vi "Parse VTG Sentence.vi"(8 "error in (no error)":errorcluster, 11 "VTG sentence":string) -> (0 "error out":errorcluster, 3 "VTG  data":T1 {"type of fix"."mode" items=["Simulator", "Not Valid", "Estimated", "Differential", "Autonomous"]})   [LabVIEW 2017, in "NMEA API.lvlib"]
doc: "Returns data contained in a particular type of NMEA sentence. The input sentence you specify must include valid NMEA formatting and end with a carriage return and line feed, or \\r\\n. You must manually select the polymorphic instance to use."
uses:
  <vilib>/robotics/Protocols/NMEA/NMEA API.lvlib
  <vilib>/robotics/Protocols/NMEA/typedefs/VTG Data.ctl
  <vilib>/robotics/Utilities/NI_Robotics Utilities.lvlib
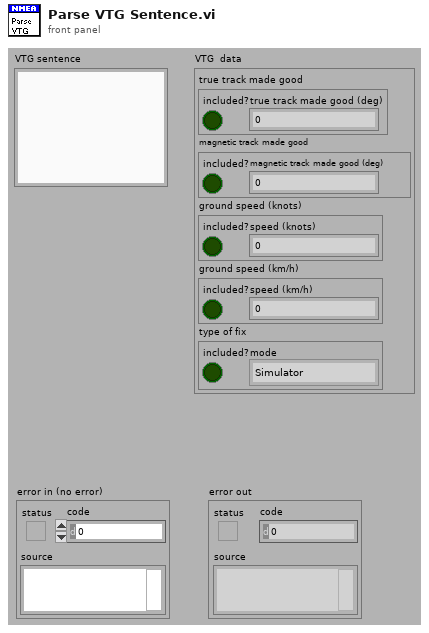
[diagram p1: front panel]
types:
  T1 = typedef "NMEA API.lvlib/VTG Data.ctl" = cluster{"true track made good":cluster{"included?":bool, "true track made good (deg)":dbl}, "magnetic track made good":cluster{"included?":bool, "magnetic track made good (deg)":dbl}, "ground speed (knots)":cluster{"included?":bool, "speed (knots)":dbl}, "ground speed (km/h)":cluster{"included?":bool, "speed (km/h)":dbl}, "type of fix":cluster{"included?":bool, "mode":u16}}
  T2 = cluster{"Boolean":bool, "True Track Made Good (Deg)":dbl}
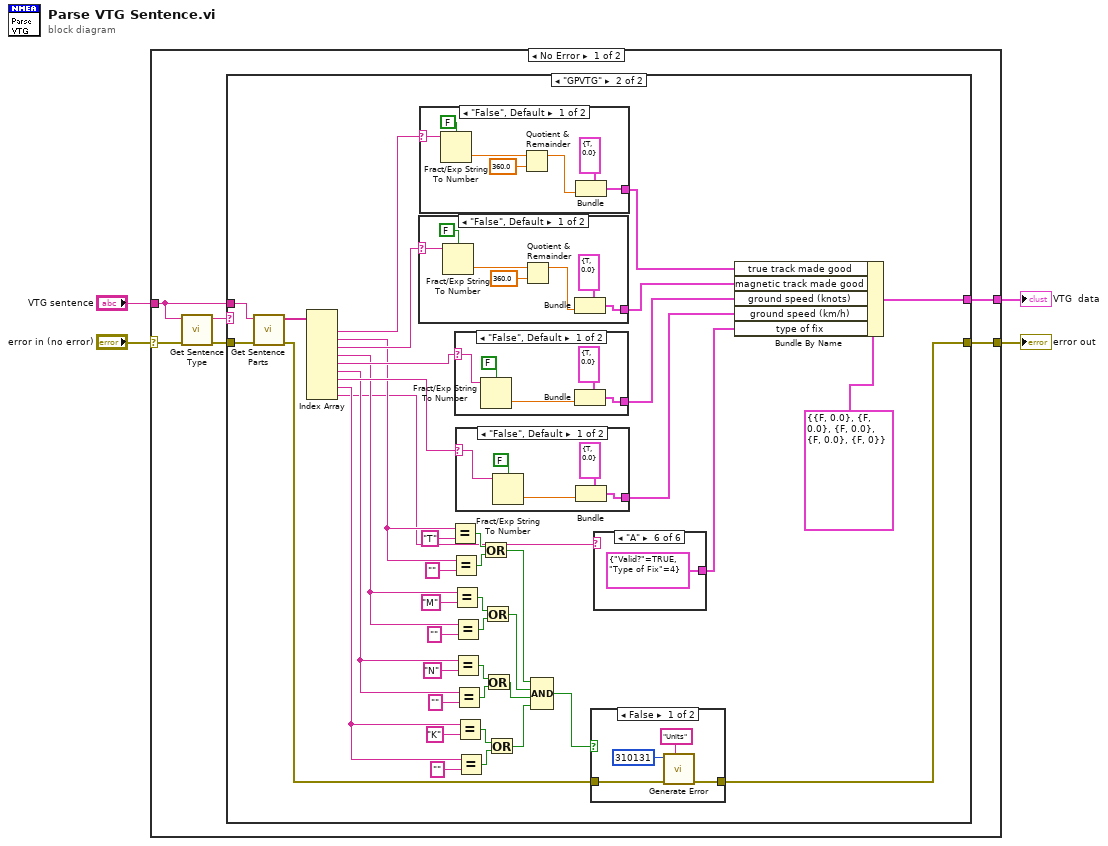
[diagram p0: block diagram]
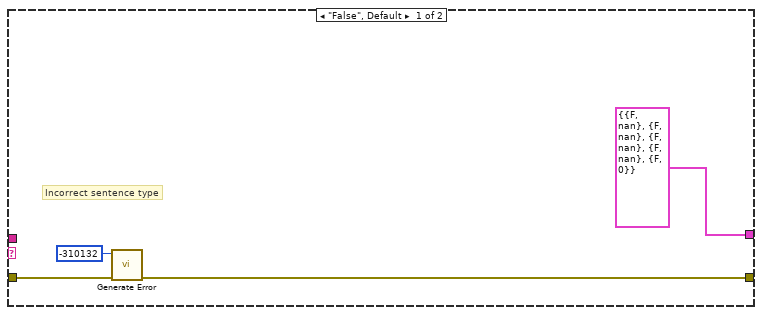
[diagram p2: hidden frame]
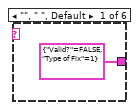
[diagram p3: hidden frame]
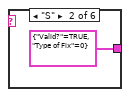
[diagram p4: hidden frame]
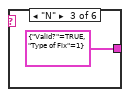
[diagram p5: hidden frame]
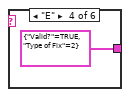
[diagram p6: hidden frame]
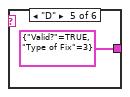
[diagram p7: hidden frame]
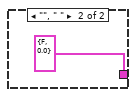
[diagram p9: hidden frame]
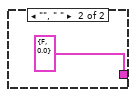
[diagram p10: hidden frame]
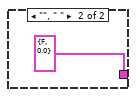
[diagram p11: hidden frame]
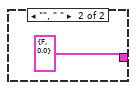
[diagram p12: hidden frame]
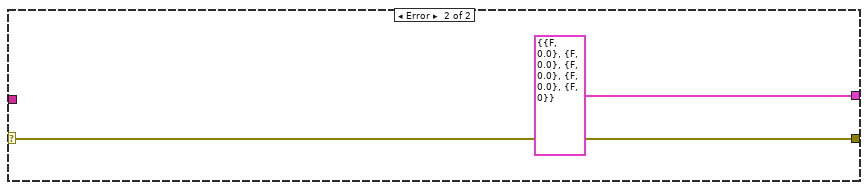
[diagram p13: hidden frame]
diagram:
  n1 = case shown="No Error" "error in (no error)" {
    selector: "error in (no error)" -> [w8 w96]
    tunnel: [w10 T1 {"true track made good"={"included?"=FALSE, "true track made good (deg)"=0.0}, "magnetic track made good"={"included?"=FALSE, "magnetic track made good (deg)"=0.0}, "ground speed (knots)"={"included?"=FALSE, "speed (knots)"=0.0}, "ground speed (km/h)"={"included?"=FALSE, "speed (km/h)"=0.0}, "type of fix"={"included?"=FALSE, "mode"=0}} ("VTG  Data")] -> w3
    tunnel: [w9 w96] -> w1
    tunnel: "VTG sentence" -> [w6 _]
    frame No Error {
      n2 = call <vilib>:"Get Sentence Type.vi"("error in (no error)"=w8, "sentence"=w6) -> ("error out"=w7:errorcluster, "sentence type"=w5:string)  [unwired: 2 in, 6 out]
      n3 = case shown="\"GPVTG\"" w5 {
        tunnel: w7 -> [w12 w56]
        tunnel: w6 -> [_ w18]
        tunnel: [T1 {"true track made good"={"included?"=FALSE, "true track made good (deg)"=nan}, "magnetic track made good"={"included?"=FALSE, "magnetic track made good (deg)"=nan}, "ground speed (knots)"={"included?"=FALSE, "speed (knots)"=nan}, "ground speed (km/h)"={"included?"=FALSE, "speed (km/h)"=nan}, "type of fix"={"included?"=FALSE, "mode"=0}} ("VTG  Data") w54] -> w10
        tunnel: [w11 w15] -> w9
        frame "False", Default {
          # "Incorrect sentence type"
          n4 = call <vilib>:"Generate Error.vi"("error in (no error)"=w12, "code"=-310132) -> ("error out"=w11:errorcluster)  [unwired: 9 in]
        }
        frame "GPVTG" {
          n5 = call <vilib>:"Get Sentence Parts.vi"("error in (no error)"=w56, "sentence"=w18) -> ("error out"=w16:errorcluster, "sentence data"=w17:string[])  [unwired: 1 in, 7 out]
          n6 = Index Array(array=w17) -> (element #1=w52:string, element #2=w29:string, element #3=w46:string, element #4=w28:string, element #5=w47:string, element #6=w27:string, element #7=w48:string, element #8=w26:string, element #9=w20:string)  [unwired: 9 in]
          n7 = case shown="\"False\", Default" w46 {
            selector: w46 -> [w84 _]
            tunnel: [w85 T2 {"Boolean"=FALSE, "True Track Made Good (Deg)"=0.0} ("True Track Made Good")] -> w51
            frame "False", Default {
              n8 = Fract/Exp String To Number(use system decimal point (T)=FALSE, string=w84) -> (number=w83:dbl)  [unwired: 3 out]
              n9 = Quotient & Remainder(x=w83, y=360.0) -> (x-y*floor(x/y)=w82:dbl)  [unwired: 1 out]
              n10 = Bundle(cluster=T2 {"Boolean"=TRUE, "True Track Made Good (Deg)"=0.0} ("True Track Made Good"), "True Track Made Good (Deg)"=w82) -> (w85:T2)  [unwired: 1 out]
            }
            frame "", " " {
            }
          }
          n11 = case shown="\"False\", Default" w52 {
            selector: w52 -> [w92 _]
            tunnel: [w93 T2 {"Boolean"=FALSE, "True Track Made Good (Deg)"=0.0} ("True Track Made Good")] -> w53
            frame "False", Default {
              n12 = Fract/Exp String To Number(use system decimal point (T)=FALSE, string=w92) -> (number=w91:dbl)  [unwired: 3 out]
              n13 = Quotient & Remainder(x=w91, y=360.0) -> (x-y*floor(x/y)=w90:dbl)  [unwired: 1 out]
              n14 = Bundle(cluster=T2 {"Boolean"=TRUE, "True Track Made Good (Deg)"=0.0} ("True Track Made Good"), "True Track Made Good (Deg)"=w90) -> (w93:T2)  [unwired: 1 out]
            }
            frame "", " " {
            }
          }
          n15 = Equal?(x=w29, y="T") -> (x = y?=w44:bool)
          n16 = Equal?(x=w29, y="") -> (x = y?=w45:bool)
          n17 = Equal?(x=w28, y="M") -> (x = y?=w39:bool)
          n18 = Equal?(x=w28, y="") -> (x = y?=w38:bool)
          n19 = Equal?(x=w27, y="N") -> (x = y?=w31:bool)
          n20 = Equal?(x=w27, y="") -> (x = y?=w30:bool)
          n21 = case shown="\"False\", Default" w47 {
            selector: w47 -> [w75 _]
            tunnel: [w76 T2 {"Boolean"=FALSE, "True Track Made Good (Deg)"=0.0} ("True Track Made Good")] -> w50
            frame "False", Default {
              n22 = Fract/Exp String To Number(use system decimal point (T)=FALSE, string=w75) -> (number=w77:dbl)  [unwired: 3 out]
              n23 = Bundle(cluster=T2 {"Boolean"=TRUE, "True Track Made Good (Deg)"=0.0} ("True Track Made Good"), "True Track Made Good (Deg)"=w77) -> (w76:T2)  [unwired: 1 out]
            }
            frame "", " " {
            }
          }
          n24 = Equal?(x=w26, y="K") -> (x = y?=w36:bool)
          n25 = case shown="\"False\", Default" w48 {
            selector: w48 -> [w69 _]
            tunnel: [w70 T2 {"Boolean"=FALSE, "True Track Made Good (Deg)"=0.0} ("True Track Made Good")] -> w49
            frame "False", Default {
              n26 = Fract/Exp String To Number(use system decimal point (T)=FALSE, string=w69) -> (number=w71:dbl)  [unwired: 3 out]
              n27 = Bundle(cluster=T2 {"Boolean"=TRUE, "True Track Made Good (Deg)"=0.0} ("True Track Made Good"), "True Track Made Good (Deg)"=w71) -> (w70:T2)  [unwired: 1 out]
            }
            frame "", " " {
            }
          }
          n28 = Equal?(x=w26, y="") -> (x = y?=w37:bool)
          n29 = Or(x=w44, y=w45) -> (x .or. y?=w25:bool)
          n30 = Or(x=w39, y=w38) -> (x .or. y?=w22:bool)
          n31 = Or(x=w31, y=w30) -> (x .or. y?=w23:bool)
          n32 = Or(x=w36, y=w37) -> (x .or. y?=w24:bool)
          n33 = Compound Arithmetic op=AND(w25, w22, w23, w24) -> (w21:bool)
          n34 = case shown="False" w21 {
            tunnel: w16 -> [w64 w67]
            tunnel: [w63 w67] -> w15
            frame False {
              n35 = call <vilib>:"Generate Error.vi"("<append> (\"\")"="Units" ("<append> (\"\")"), "error in (no error)"=w64, "code"=310131) -> ("error out"=w63:errorcluster)  [unwired: 8 in]
            }
            frame True {
            }
          }
          n36 = case shown="\"A\"" w20 {
            tunnel: [cluster{"Valid?":bool, "Type of Fix":u16} {"Valid?"=FALSE, "Type of Fix"=1} ("Type of Fix") cluster{"Valid?":bool, "Type of Fix":u16} {"Valid?"=TRUE, "Type of Fix"=0} ("Type of Fix") cluster{"Valid?":bool, "Type of Fix":u16} {"Valid?"=TRUE, "Type of Fix"=1} ("Type of Fix") cluster{"Valid?":bool, "Type of Fix":u16} {"Valid?"=TRUE, "Type of Fix"=2} ("Type of Fix") cluster{"Valid?":bool, "Type of Fix":u16} {"Valid?"=TRUE, "Type of Fix"=3} ("Type of Fix") cluster{"Valid?":bool, "Type of Fix":u16} {"Valid?"=TRUE, "Type of Fix"=4} ("Type of Fix")] -> w19
            frame "", " ", Default {
            }
            frame "S" {
            }
            frame "N" {
            }
            frame "E" {
            }
            frame "D" {
            }
            frame "A" {
            }
          }
          n37 = Bundle By Name(cluster=T1 {"true track made good"={"included?"=FALSE, "true track made good (deg)"=0.0}, "magnetic track made good"={"included?"=FALSE, "magnetic track made good (deg)"=0.0}, "ground speed (knots)"={"included?"=FALSE, "speed (knots)"=0.0}, "ground speed (km/h)"={"included?"=FALSE, "speed (km/h)"=0.0}, "type of fix"={"included?"=FALSE, "mode"=0}} ("VTG  Data"), "true track made good"=w53, "magnetic track made good"=w51, "ground speed (knots)"=w50, "ground speed (km/h)"=w49, "type of fix"=w19) -> (w54:T1)
        }
      }
    }
    frame Error {
    }
  }
  "error out" <- w1
  "VTG  data" <- w3
